vi "Waterfall Mode Read.vi"(4 "error in (no error)":errorcluster, 6 "Container State":T3, 7 "Display State In":T1) -> (0 "error out":errorcluster, 2 "Value":enum16{"Lines", "Slices"}(ring), 3 "Display State Out":T1)   [LabVIEW 2017, in "3D Waterfall.xctl"]
uses:
  <vilib>/Math Plots/3D Math Plots/3D Waterfall/3D Waterfall XCtrl/3D Waterfall.xctl
  <vilib>/_xctls/Container State.ctl
  <vilib>/Math Plots/3D Math Plots/3D Waterfall/3D Waterfall XCtrl/State.ctl
  <vilib>/Math Plots/3D Math Plots/3D Waterfall/3D Waterfall/3D Waterfall.lvclass
  e:/builds/penguin/labview/branches/2017/dev/dist/vi.lib/Math Plots/3D Math Plots/3D Plot/3D Plot/3D Plot.lvclass
  <vilib>/Math Plots/3D Math Plots/3D Plot/Action String/3DMathPlot Ctrl Act Queue.ctl
  <vilib>/Math Plots/3D Math Plots/3D Plot/Action String/3DMathPlot Ctrl Act Cluster.ctl
  <vilib>/Math Plots/3D Math Plots/3D Plot/Action String/3DMathPlot State Class.ctl
  <vilib>/Math Plots/3D Math Plots/3D Plot/3D Plot/3D Plot.lvclass
  <vilib>/_xctls/XControlSupport.lvlib
panel:
  # "Replace the Value Indicator below with an Indicator of desired type.\nDo not remove this Indicator or the others from the connector pane. \nDo not change the connector pane pattern.\nThe Value Indicator should always be the second terminal from top on the output side in the connector pane."
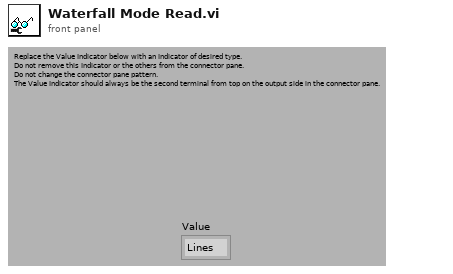
[diagram p1: front panel]
types:
  T1 = typedef "3D Waterfall.xctl/State.ctl" = cluster{"3D Waterfall.lvclass":refnum<class "3D Waterfall.lvclass">, "Control Ref Queue":T2, "Main Frame Color":u32, "Ramp Palette Color":u32, "Projection Palette Color":u32}
  T2 = typedef "3DMathPlot Ctrl Act Queue.ctl" = refnum<queue>
  T3 = typedef "XControlSupport.lvlib/Container State.ctl" = cluster{"Indicator?":bool, "Run Mode?":bool, " Refnum":refnum<vi>}
  T4 = typedef "3D Waterfall.lvclass/3D Waterfall Propery Array.ctl" = T5[]
  T5 = typedef "3D Waterfall.lvclass/3D Waterfall Property.ctl" = cluster{"General Property":cluster{"Plot Name":string, "Coordinate System":enum16{"Cartesian", "Cylindrical", "Spherical"}, "Opacity":sgl}, "Projection Property":cluster{"Draw XY":bool, "Draw YZ":bool, "Draw XZ":bool}, "Plot Property":cluster{"Line Style":T6, "Line Width":sgl, "Color Ramp Cluster":T7, "Antialiasing":bool}, "Waterfall Property":cluster{"Waterfall Mode":enum16{"Lines", "Slices"}}}
  T6 = typedef "3D Plot.lvclass/Line Type.ctl" = enum16{"None", "Solid", "Dash", "Dot", "Dash Dot"}
  T7 = typedef "3D Plot.lvclass/Color Ramp Cluster.ctl" = cluster{"Color Ramp Style":enum16{"None", "Shaded", "Color spectrum", "Grey scale", "Custom"}, "Color Ramp Array":u32[], "Color Ramp Index":i32[], "Interpolate?":bool, "Logarithm?":bool}
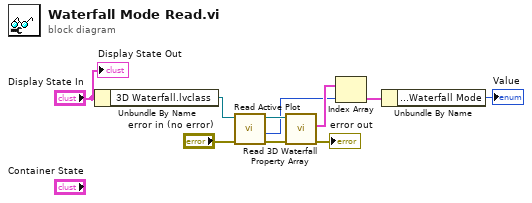
[diagram p0: block diagram]
diagram:
  n1 = Unbundle By Name("Display State In") -> ("3D Waterfall.lvclass"=w9:refnum<class "3D Waterfall.lvclass">)
  n2 = call <vilib>:"Read Active Plot.vi"("error in (no error)"="error in (no error)", "3D Plot.lvclass in"=w9) -> ("error out"=w6:errorcluster, "Active Plot"=w5:i32, "3D Plot.lvclass out"=w8:refnum<class "3D Waterfall.lvclass">)  [unwired: 7 out]
  n3 = call <vilib>:"Read 3D Waterfall Property Array.vi"("error in (no error)"=w6, "3D Waterfall.lvclass in"=w8) -> ("error out"=→"error out":errorcluster, "3D Waterfall Property Array"=w7:T4)  [unwired: 8 out]
  n4 = Index Array(array=w7, index=w5) -> (element=w10:T5)
  n5 = Unbundle By Name(w10) -> ("Waterfall Property.Waterfall Mode"=→"Value":enum16{"Lines", "Slices"})
  "Display State Out" <- "Display State In"
